vi "error test.vi"() -> ()   [LabVIEW 2014]
panel:
  out "testErr":string
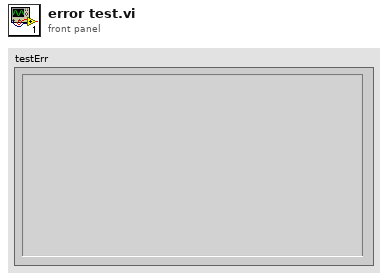
[diagram p1: front panel]
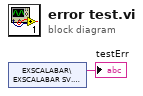
[diagram p0: block diagram]
diagram:
  n1 = shared-variable "EXSCALABAR\\EXSCALABAR SV.lvlib\\testErr"() -> (→"testErr":string)  [unwired: 1 in, 1 out]
